vi "Analog Input (FPGA).vi"() -> ()   [LabVIEW 2014]
doc: "This VI will continually read single point values from 4 channels of an analog input module at a specified rate."
uses:
  <vilib>/rvi/Emulation/niFpgaGetClockAttributes.vi
  <vilib>/rvi/Emulation/niFpgaSctlEmulationGetInTimedLoop.vi
  <vilib>/rvi/Emulation/niFpgaEmulationReportErrorSimple.vi
  <vilib>/rvi/eio/common/nirviEmuTemplateMethod_errors.vi
  <vilib>/rvi/Emulation/niFpgaCriticalErrorInLSC.vi
  <vilib>/eio/EIONode/EIONode.xnode
panel:
  out "output cluster":T1
  in  "stop":bool
  out "FPGA Error Out":errorcluster
  # "For instructions, and select Help>>Show Context Help and hover over the icon."
  # "Output Parameters"
  # "Input Parameters"
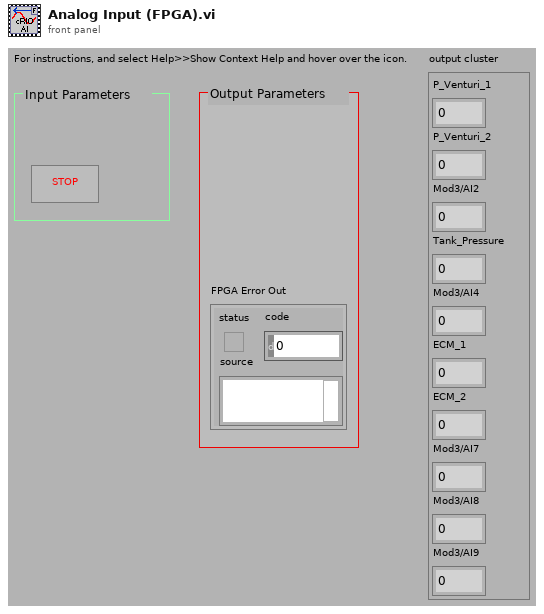
[diagram p1: front panel]
types:
  T1 = cluster{"P_Venturi_1":fxp<+/-,26,5>, "P_Venturi_2":fxp<+/-,26,5>, "Mod3/AI2":fxp<+/-,26,5>, "Tank_Pressure":fxp<+/-,26,5>, "Mod3/AI4":fxp<+/-,26,5>, "ECM_1":fxp<+/-,26,5>, "ECM_2":fxp<+/-,26,5>, "Mod3/AI7":fxp<+/-,26,5>, "Mod3/AI8":fxp<+/-,26,5>, "Mod3/AI9":fxp<+/-,26,5>}
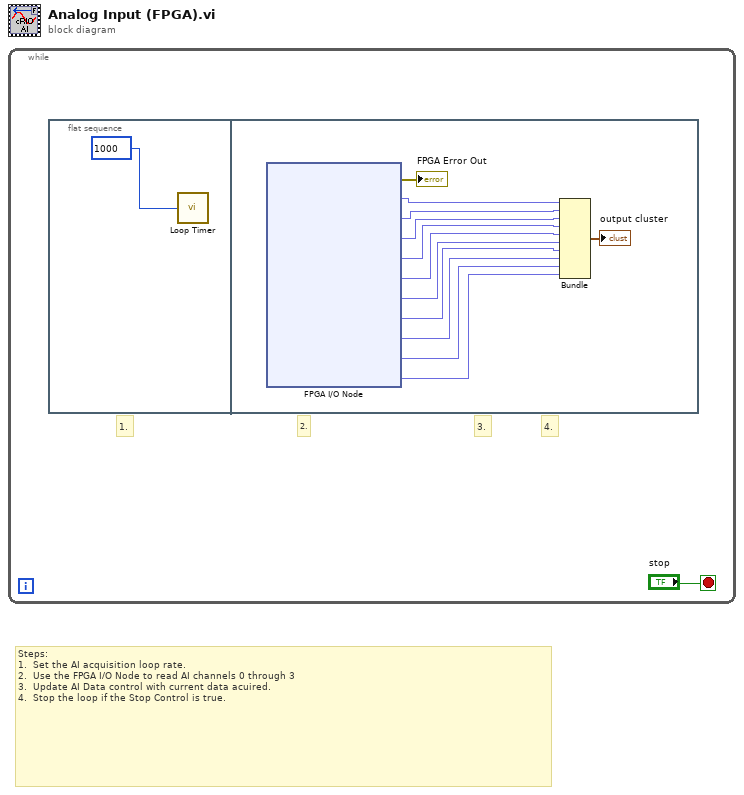
[diagram p0: block diagram]
diagram:
  # "Steps: \n1.  Set the AI acquisition loop rate.\n2.  Use the FPGA I/O Node to read AI channels 0 through 3\n3.  Update AI Data control with current data acuired.\n4.  Stop the loop if the Stop Control is true."
  n1 = while {
    stop <- "stop" stop-if-true
    # "4."
    # "3."
    # "2."
    # "1."
    n2 = flat-sequence {
      frame #0 {
        n3 = call "Loop Timer"("Count(mSec)"=u32 1000 ("AI Sample Rate(uSec)")) -> ()  [unwired: 1 out]
      }
      frame #1 {
        n4 = xnode "FPGA I/O Node"() -> ("error out"=→"FPGA Error Out":errorcluster, "P_Venturi_1"=w13:fxp<+/-,26,5>, "P_Venturi_2"=w12:fxp<+/-,26,5>, "Mod3/AI2"=w11:fxp<+/-,26,5>, "Tank_Pressure"=w10:fxp<+/-,26,5>, "Mod3/AI4"=w9:fxp<+/-,26,5>, "ECM_1"=w8:fxp<+/-,26,5>, "ECM_2"=w7:fxp<+/-,26,5>, "Mod3/AI7"=w6:fxp<+/-,26,5>, "Mod3/AI8"=w5:fxp<+/-,26,5>, "Mod3/AI9"=w4:fxp<+/-,26,5>)  [unwired: 11 in, 10 out]
        n5 = Bundle("P_Venturi_1"=w13, "P_Venturi_2"=w12, "Mod3/AI2"=w11, "Tank_Pressure"=w10, "Mod3/AI4"=w9, "ECM_1"=w8, "ECM_2"=w7, "Mod3/AI7"=w6, "Mod3/AI8"=w5, "Mod3/AI9"=w4) -> (→"output cluster":T1)  [unwired: 1 out]
      }
    }
  }
